vi "SUBVISEMAFORTRAINER.vi"() -> ()   [LabVIEW 2024]
panel:
  in  "stop":bool
  out "Verde Pietoni":bool
  out "Rosu Pietoni":bool
  out "Verde":bool
  out "Galben":bool
  out "Rosu":bool
  in  "Vehicule de urgenta":bool
  in  "Numar Vehicule":dbl
  in  "Numar Pietoni":dbl
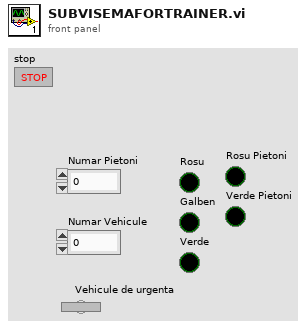
[diagram p1: front panel]
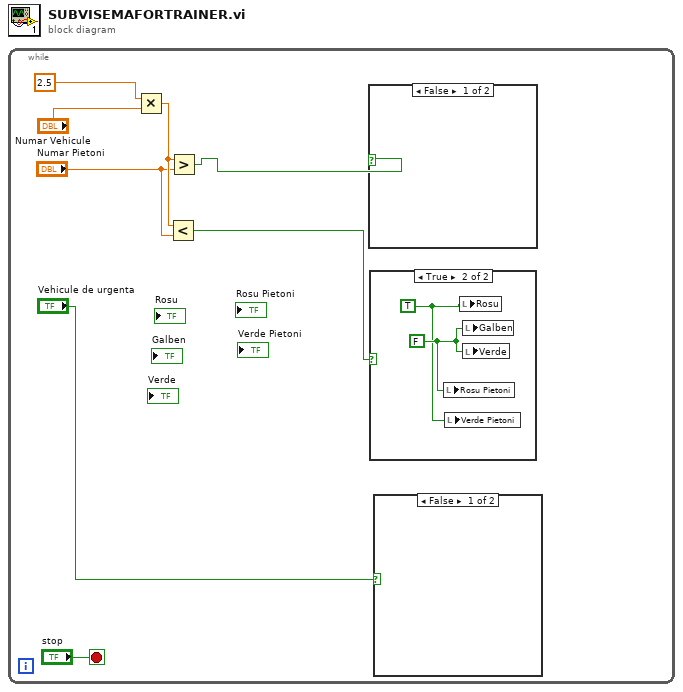
[diagram p0: block diagram]
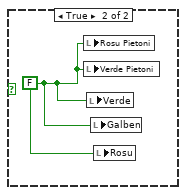
[diagram p2: hidden frame]
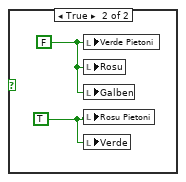
[diagram p4: hidden frame]
diagram:
  n1 = while {
    stop <- "stop" stop-if-true
    n2 = Multiply(x=2.5, y="Numar Vehicule") -> (x*y=w6:dbl)
    n3 = Less?(x=w6, y="Numar Pietoni") -> (x < y?=w1:bool)
    n4 = Greater?(x=w6, y="Numar Pietoni") -> (0:w3:bool)
    n5 = case shown="False" w3 {
      frame False {
      }
      frame True {
        w12 = TRUE ("Rosu Pietoni")
        w13 = FALSE ("Verde Pietoni")
        n6 = local write "Verde Pietoni"(w13) -> ()
        n7 = local write "Rosu"(w13) -> ()
        n8 = local write "Galben"(w13) -> ()
        n9 = local write "Rosu Pietoni"(w12) -> ()
        n10 = local write "Verde"(w12) -> ()
      }
    }
    n11 = case shown="True" w1 {
      frame False {
      }
      frame True {
        w11 = FALSE ("Galben")
        w10 = TRUE ("Rosu")
        n12 = local write "Rosu Pietoni"(w11) -> ()
        n13 = local write "Verde Pietoni"(w10) -> ()
        n14 = local write "Rosu"(w10) -> ()
        n15 = local write "Galben"(w11) -> ()
        n16 = local write "Verde"(w11) -> ()
      }
    }
    n17 = case shown="False" "Vehicule de urgenta" {
      frame False {
      }
      frame True {
        w9 = FALSE ("Rosu")
        n18 = local write "Rosu Pietoni"(w9) -> ()
        n19 = local write "Verde Pietoni"(w9) -> ()
        n20 = local write "Verde"(w9) -> ()
        n21 = local write "Galben"(w9) -> ()
        n22 = local write "Rosu"(w9) -> ()
      }
    }
  }
